vi "Reverse Convert Stroker Value.vi"(9 "Variable":T1, 10 "Value in":dbl) -> (2 "Converted value":dbl)   [LabVIEW 2011]
uses:
  Tool/Variable List Tool Analog.ctl
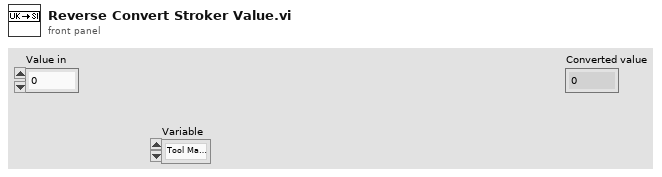
[diagram p1: front panel]
types:
  T1 = typedef "Variable List Tool Analog.ctl" = enum16{"Tool Max Temperature", "Tool (Controller) Temperature", "Tool Supply Voltage", "Tool (Controller) Current", "Tool Acceleration X", "Tool Acceleration Y", "Tool Acceleration Z", "Tool Acceleration Sum", "Tool Inclination", "Tool Rotation", "Tool GP Sensor 1", "Tool GP Sensor 2", "Tool (Pressure 1) Temperature", "Tool Pressure 1 RAW", "Tool (Pressure 2) Temperature", "Tool Pressure 2 RAW", "Tool (Solenoid) Temperature", "Tool Solenoid Position", "PSU Temp", "Head Voltage", "PSU Main Voltage out", "PSU Main Current out", "Upper Tension Sub Temp", "Tool Upper Tension Sub Raw", "Lower Tension Sub Temp", "Tool Lower Tension Sub Raw", "Tool Var27 - Reserved", "Tool Var28 - Reserved", "Tool Var29 - Reserved", "Tool Var30 - Reserved", "Stroke Extension", "Stroke In Force", "Stroke Out Force", "Stroke Force", "Stroker Pressure 1", "Stroker Pressure 2", "Stroker Upper Tension Sub", "Stroker Lower Tension Sub", "Stroker Var09 - Reserved", "Stroker Var10 - Reserved", "Tractor Upper Tension Sub", "Tractor Lower Tension Sub", "Tractor Var03 - Reserved", "Tractor Var04 - Reserved", "Tool Temperature sensor", "Tool Motor Voltage", "Tool Motor Current", "Tool Motor Torque", "Tool weight on bit", "Tool Motor RPM"}
  T2 = typedef "Fixed Analog Channel Definition.ctl" = cluster{"ID":u16, "Name":string, "Quantity":T3, "Unit":string, "Maximum upd":T4, "Comment":string, "Help file Name":string, "Help file Section ":string, "Category":T5, "User adjustable Scaling":bool, "Default Scaling":T6, "Default Unit":i32, "Classification":T7}
  T3 = typedef "Quantity enum.ctl" = enum16{"NA", "Acceleration", "Angle", "Current", "Force", "Distance", "Pressure", "Resistance", "Rotational Speed", "Speed", "Temperature", "Tension", "Torque", "Voltage", "Weight"}
  T4 = typedef "Update frequensies.ctl" = enum16{"2 Hz", "1 Hz", "0.1 Hz"}
  T5 = typedef "Channel catagory Enum.ctl" = enum16{"No Category", "Power", "Temperature", "Pressure"}
  T6 = typedef "Scaling.ctl" = cluster{"Gain":dbl, "Offset":dbl}
  T7 = typedef "Channel Classification Enum.ctl" = enum16{"Basic", "Advanced", "Expert", "Unused"}
  T8 = typedef "User Setting Analog Channel Bg.ctl" = cluster{"Scaling":T6, "Limits and responces":T9, "Allow Graph selection by user":bool, "Unit":u16}
  T9 = typedef "Alarm Setup Analog.ctl" = cluster{"Technical Error(NA)":T10, "LL":T10, "L":T10, "H":T10, "HH":T10, "Limits":T12}
  T10 = typedef "Alarm Responce.ctl" = cluster{"Action":T11, "Alarm":bool}
  T11 = typedef "Action List.ctl" = enum16{"No Action", "Stop Motor", "Turn Off HV"}
  T12 = typedef "Limits.ctl" = cluster{"LL":dbl, "L":dbl, "H":dbl, "HH":dbl}
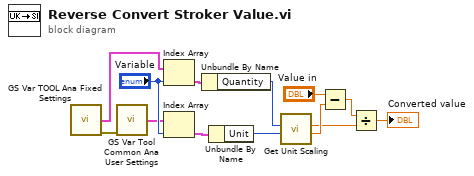
[diagram p0: block diagram]
diagram:
  n1 = call "GS Var TOOL Ana Fixed Settings.vi"() -> ("Tool Analog var Fixed out"=w7:T2[], "error out"=w12:errorcluster)  [unwired: 13 in, 1 out]
  n2 = call "GS Var Tool Common Ana User Settings.vi"("error in (no error)"=w12) -> ("Tool Analog var User settigns out"=w6:T8[])  [unwired: 12 in, 2 out]
  n3 = Index Array(array=w7, index="Variable") -> (element=w9:T2)
  n4 = Index Array(array=w6, index="Variable") -> (element=w8:T8)
  n5 = Unbundle By Name(w9) -> ("Quantity"=w10:T3)
  n6 = Unbundle By Name(w8) -> ("Unit"=w11:u16)
  n7 = call "Get Unit Scaling.vi"("Unit Index"=w11, "Quantity"=w10) -> ("Offset"=w4:dbl, "Gain"=w2:dbl)  [unwired: 7 in, 1 out]
  n8 = Subtract(x="Value in", y=w4) -> (x-y=w3:dbl)
  n9 = Divide(x=w3, y=w2) -> (x/y=→"Converted value":dbl)
